vi "cameraSettingsGlobalF.vi"(9 "PixelflySettings":refnum<class "PixelflySettings.lvclass">, 10 "Action":enum16{"Write", "Read"}(ring)) -> (1 "PixelflySettings":refnum<class "PixelflySettings.lvclass">)   [LabVIEW 2009, in "Tools.lvlib" / "Settings.lvlib"]
uses:
  Settings.lvlib
  PixelFlySettings/PixelflySettings.lvclass
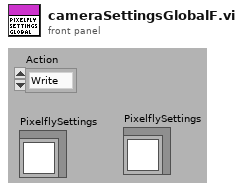
[diagram p1: front panel]
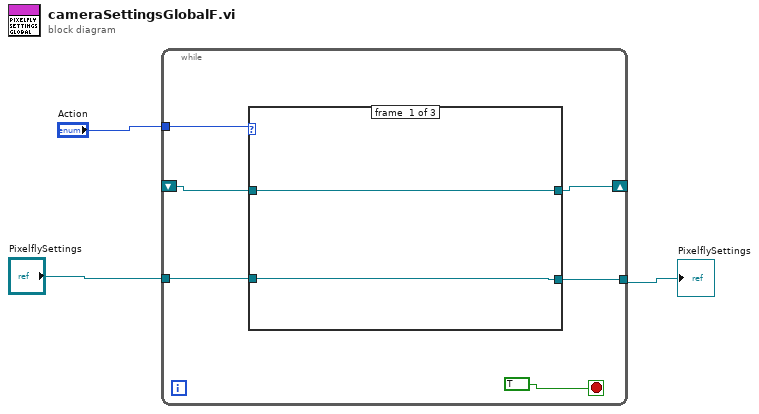
[diagram p0: block diagram]
diagram:
  n1 = while {
    tunnel: "Action" -> [w9]
    shift-right: [w4] -> _
    shift-left: _ -> [w6]
    tunnel: "PixelflySettings" -> [w7]
    tunnel: [w5] -> w1
    stop <- TRUE stop-if-true
    n2 = case shown="\"Read\"" w9 {
      tunnel: [w11 w12 w13] -> w4
      tunnel: w7 -> [w10 w12 _]
      tunnel: w6 -> [w11 _ w13]
      tunnel: [w10 w12 w13] -> w5
      frame #0 {
      }
      frame #1 {
      }
      frame #2 {
      }
    }
  }
  "PixelflySettings" <- w1
